vi "write path.vi"(8 "error in (no error)":errorcluster, 10 "Path Cluster":T2, 11 "Stepper in":refnum<class "Stepper.lvclass">) -> (0 "error out":errorcluster, 3 "Stepper out":refnum<class "Stepper.lvclass">)   [LabVIEW 2025, in "Motor.lvlib" / "Stepper.lvclass"]
uses:
  Stepper.lvclass
  Path Mode.ctl
  Stepper.lvclass/Stepper.ctl
  Motor.lvlib
panel:
  out "appended array":u32[](array[numeric])
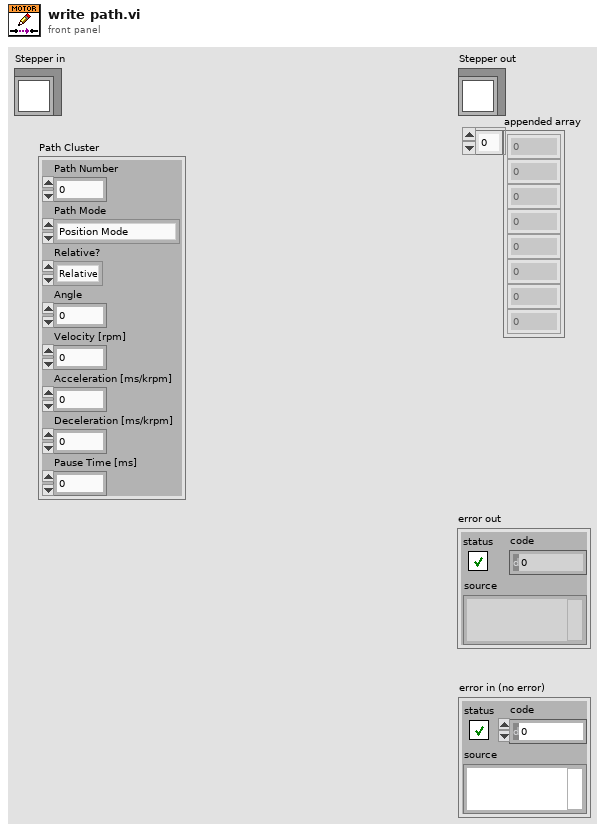
[diagram p1: front panel]
types:
  T1 = typedef "Motor.lvlib/Path Mode.ctl" = enum16{"Position Mode", "Velocity Mode", "Homing Mode"}
  T2 = cluster{"Path Number":i32, "Path Mode":T1, "Relative?":enum16{"Relative", "Absolute"}, "Angle":dbl, "Velocity [rpm]":i32, "Acceleration [ms/krpm]":i32, "Deceleration [ms/krpm]":i32, "Pause Time [ms]":i32}
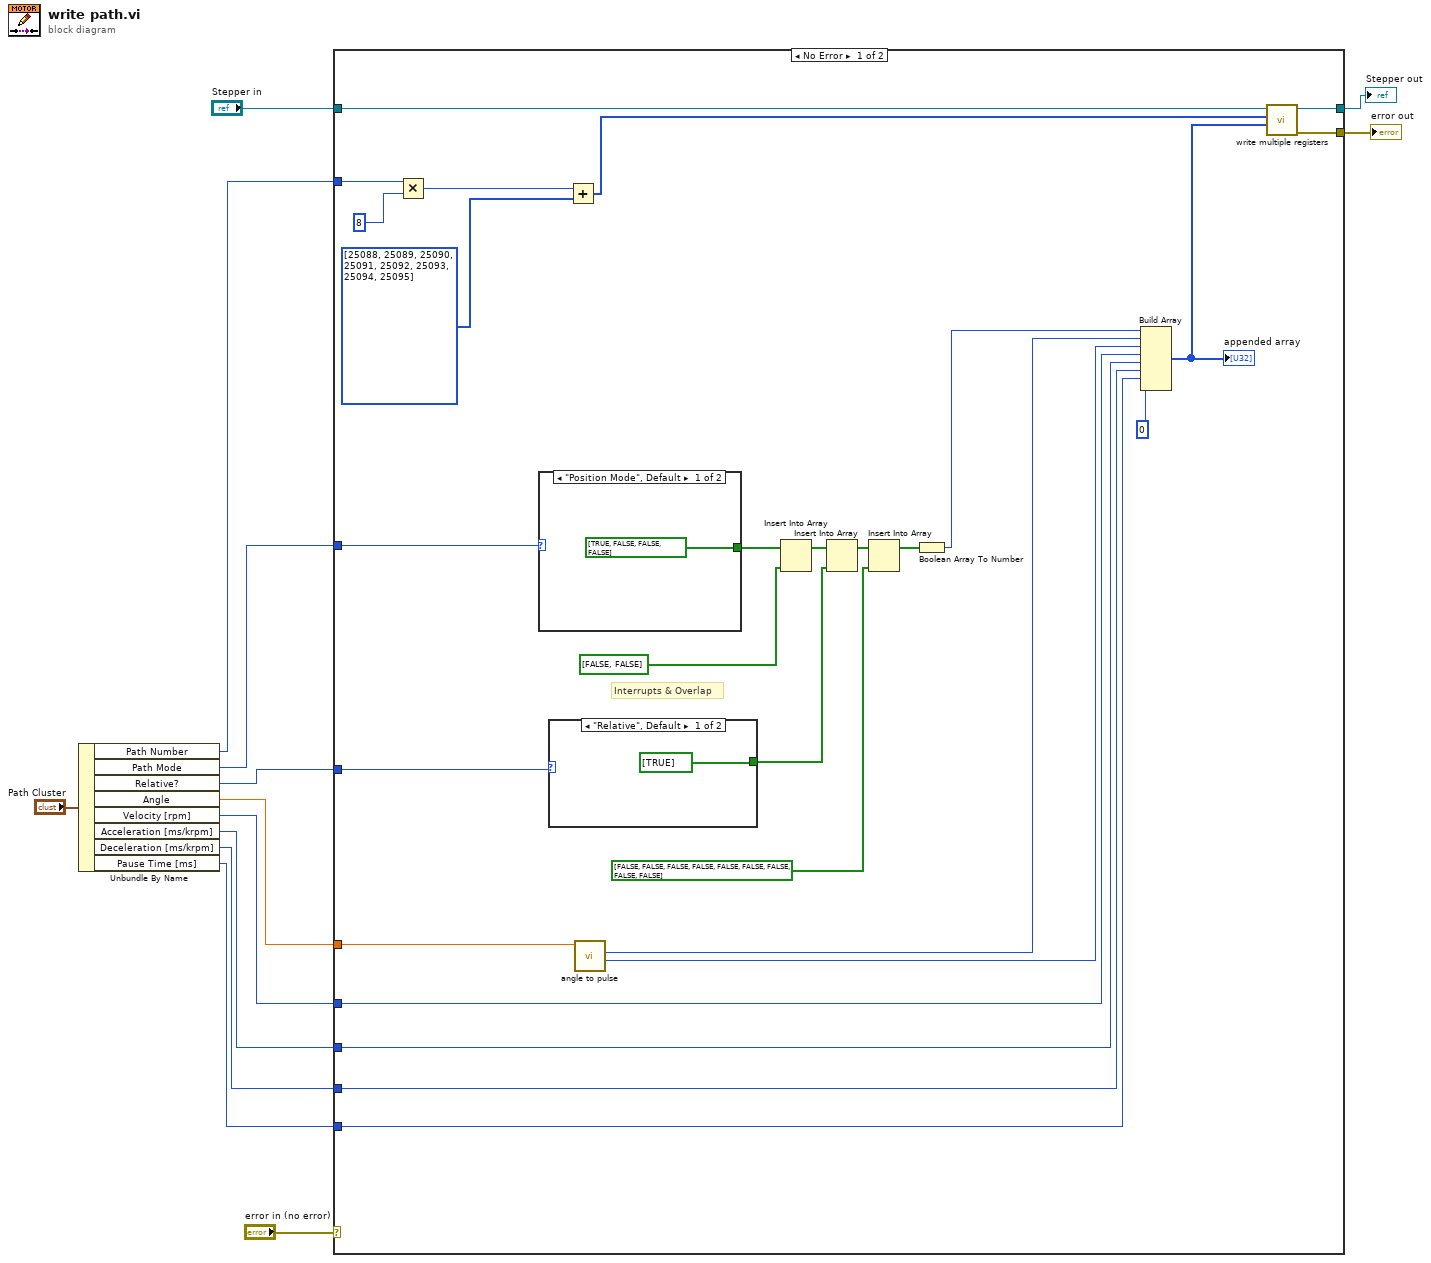
[diagram p0: block diagram]
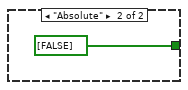
[diagram p2: hidden frame]
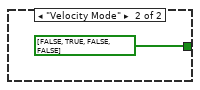
[diagram p3: hidden frame]
diagram:
  n1 = Unbundle By Name("Path Cluster") -> ("Path Number"=w8:i32, "Path Mode"=w7:T1, "Relative?"=w6:enum16{"Relative", "Absolute"}, "Angle"=w5:dbl, "Velocity [rpm]"=w4:i32, "Acceleration [ms/krpm]"=w3:i32, "Deceleration [ms/krpm]"=w2:i32, "Pause Time [ms]"=w1:i32)
  n2 = case shown="No Error" "error in (no error)" {
    selector: "error in (no error)" -> [_ w46]
    tunnel: [w14 w46] -> w12
    tunnel: [w39 w45] -> w10
    tunnel: "Stepper in" -> [w40 w45]
    tunnel: w8 -> [w38 _]
    tunnel: w7 -> [w33 _]
    tunnel: w6 -> [w32 _]
    tunnel: w5 -> [w18 _]
    tunnel: w4 -> [w23 _]
    tunnel: w3 -> [w22 _]
    tunnel: w2 -> [w21 _]
    tunnel: w1 -> [w20 _]
    frame No Error {
      # "Interrupts & Overlap"
      n3 = Multiply(x=w38, y=8) -> (x*y=w36:i32)
      n4 = case shown="\"Position Mode\", Default" w33 {
        tunnel: [bool[] [TRUE, FALSE, FALSE, FALSE] bool[] [FALSE, TRUE, FALSE, FALSE]] -> w31
        frame "Position Mode", Default {
        }
        frame "Velocity Mode" {
        }
      }
      n5 = case shown="\"Relative\", Default" w32 {
        tunnel: [bool[] [TRUE] bool[] [FALSE]] -> w28
        frame "Relative", Default {
        }
        frame "Absolute" {
        }
      }
      n6 = Add(x=w36, y=u16[] [25088, 25089, 25090, 25091, 25092, 25093, 25094, 25095] ("addresses")) -> (x+y=w34:i32[])
      n7 = call "angle to pulse.vi"("Angle"=w18) -> ("lo(x)"=w16:u16, "hi(x)"=w17:u16)  [unwired: 8 in, 1 out]
      n8 = Insert Into Array(array=w31, new element=bool[] [FALSE, FALSE]) -> (w29:bool[])  [unwired: 1 in]
      n9 = Insert Into Array(array=w29, new element=w28) -> (w27:bool[])  [unwired: 1 in]
      n10 = Insert Into Array(array=w27, new element=bool[] [FALSE, FALSE, FALSE, FALSE, FALSE, FALSE, FALSE, FALSE, FALSE]) -> (w25:bool[])  [unwired: 1 in]
      n11 = Boolean Array To Number(Boolean array=w25) -> (number=w24:u32)
      n12 = Build Array(w24, w17, w16, w23, w22, w21, w20, u32 0 ("element")) -> (w15:u32[])
      "appended array" <- w15
      n13 = call-dynamic "write multiple registers.vi"("register values"=w15, "addresses"=w34, "Stepper in"=w40) -> ("error out"=w14:errorcluster, "Stepper out"=w39:refnum<class "Stepper.lvclass">)  [unwired: 7 in]
    }
    frame Error {
    }
  }
  "error out" <- w12
  "Stepper out" <- w10
